vi "Sweep iteration instruction generator with starting step (SubVI).vi"(5 "Sweep plane & fixed axis":string, 6 "Sweep starts later":i32, 7 "Octant":string, 8 "Angle theta [degrees]":dbl, 9 "Magnetic field strength [µT]":dbl, 10 "Number of steps":dbl, 11 "Current iteration":i32) -> (0 "Magnetic field z [µT]":dbl, 1 "Magnetic field y [µT]":dbl, 2 "Magnetic field x [µT]":dbl, 3 "Azimuthal angle \"phi\"":dbl, 4 "Output string instruction":string)   [LabVIEW 2018]
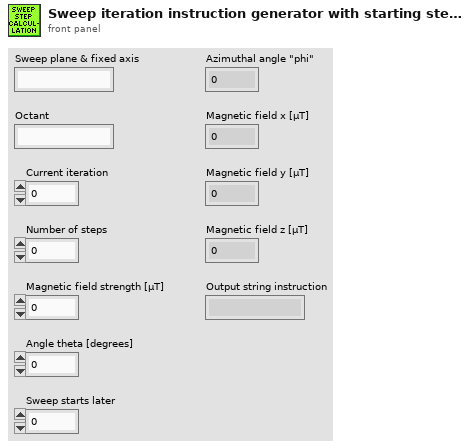
[diagram p1: front panel]
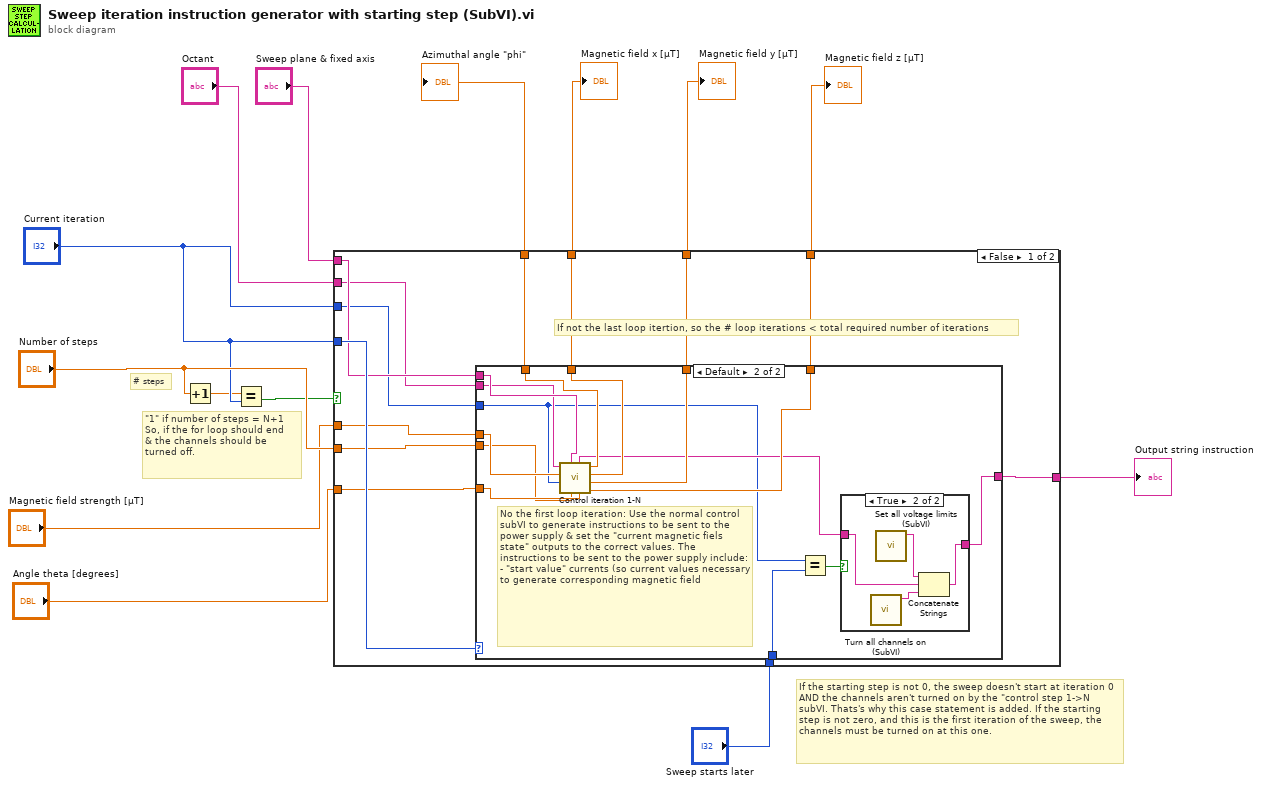
[diagram p0: block diagram]
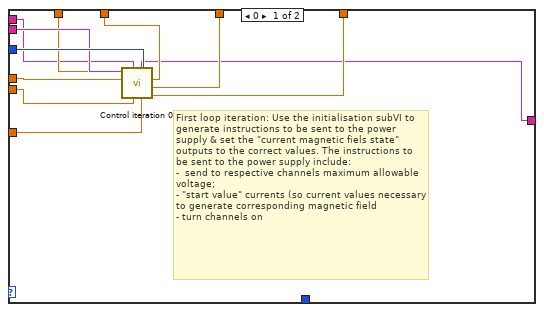
[diagram p2: hidden frame]
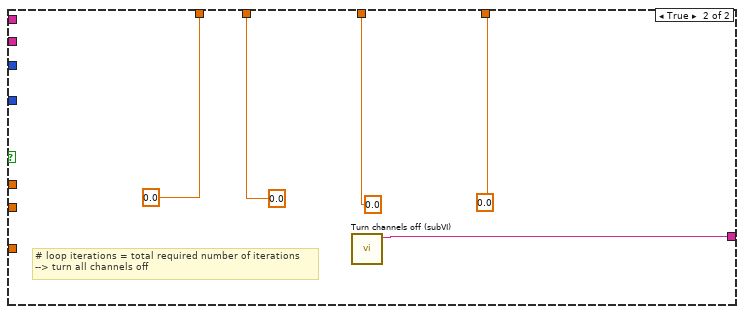
[diagram p4: hidden frame]
diagram:
  # "If the starting step is not 0, the sweep doesn't start at iteration 0 AND the channels aren't turned on by the \"control step 1->N subVI. Thats's why this case statement is added. If the starting step is not zero, and this is the first iteration of the sweep, the channels must be turned on at this one."
  # "\"1\" if number of steps = N+1\nSo, if the for loop should end \n& the channels should be \nturned off."
  # "# steps"
  n1 = Increment(x="Number of steps") -> (x+1=w1:dbl)
  n2 = Equal?(x=w1, y="Current iteration") -> (x = y?=w11:bool)
  n3 = case shown="False" w11 {
    tunnel: [w20 0.0 ("Azimuthal angle \"phi\"")] -> w10
    tunnel: [w17 0.0 ("Magnetic field x [µT]")] -> w6
    tunnel: [w19 0.0 ("Magnetic field y [µT]")] -> w5
    tunnel: [w18 0.0 ("Magnetic field z [µT]")] -> w4
    tunnel: "Current iteration" -> [w27 _]
    tunnel: "Sweep plane & fixed axis" -> [w26 _]
    tunnel: "Octant" -> [w25 _]
    tunnel: "Magnetic field strength [µT]" -> [w24 _]
    tunnel: "Current iteration" -> [w23 _]
    tunnel: "Number of steps" -> [w22 _]
    tunnel: "Angle theta [degrees]" -> [w21 _]
    tunnel: [w16 w58] -> w3
    tunnel: "Sweep starts later" -> [w15 _]
    frame False {
      # "If not the last loop itertion, so the # loop iterations < total required number of iterations"
      n4 = case shown="Default" w27 {
        tunnel: w26 -> [w29 w52]
        tunnel: w25 -> [w33 w51]
        tunnel: w24 -> [w38 w50]
        tunnel: w23 -> [w37 w40]
        tunnel: w22 -> [w28 w44]
        tunnel: w21 -> [w36 w49]
        tunnel: [w30 w48] -> w20
        tunnel: [w32 w47] -> w17
        tunnel: [w34 w46] -> w19
        tunnel: [w35 w45] -> w18
        tunnel: [w31 w41] -> w16
        tunnel: w15 -> [_ w43]
        frame 0 {
          # "First loop iteration: Use the initialisation subVI to generate instructions to be sent to the power supply & set the \"current magnetic fiels state\" outputs to the correct values. The instructions to be sent to the power supply include:\n-  send to respective channels maximum allowable voltage;\n- \"start value\" currents (so current values necessary to generate corresponding magnetic field \n- turn channels on"
          n5 = call "Control iteration 0.vi"("Angle theta [degrees]"=w36, "Number of steps"=w28, "Sweep plane & fixed axis"=w29, "Current iteration"=w37, "Magnetic field strength [µT]"=w38, "Octant"=w33) -> ("Magnetic field z [µT]"=w35:dbl, "Magnetic field y [µT]"=w34:dbl, "Magnetic field x [µT]"=w32:dbl, "Current angle"=w30:dbl, "Output instructions iteration 0"=w31:string)  [unwired: 1 in]
        }
        frame Default {
          # "No the first loop iteration: Use the normal control subVI to generate instructions to be sent to the power supply & set the \"current magnetic fiels state\" outputs to the correct values. The instructions to be sent to the power supply include:\n- \"start value\" currents (so current values necessary to generate corresponding magnetic field"
          n6 = call "Control iteration 1-N.vi"("Angle theta [degrees]"=w49, "Number of steps"=w44, "Sweep plane & fixed axis"=w52, "Current iteration"=w40, "Magnetic field strength [µT]"=w50, "Octant"=w51) -> ("Magnetic field z [µT]"=w45:dbl, "Magnetic field y [µT]"=w46:dbl, "Magnetic field x [µT]"=w47:dbl, "Current angle"=w48:dbl, "Output instructions 1->N"=w42:string)  [unwired: 1 in]
          n7 = Equal?(x=w40, y=w43) -> (x = y?=w39:bool)
          n8 = case shown="True" w39 {
            tunnel: w42 -> [w53 w56]
            tunnel: [w53 w54] -> w41
            frame False {
            }
            frame True {
              n9 = call "Turn all channels on (SubVI).vi"() -> ("String"=w57:string)  [unwired: 11 in]
              n10 = call "Set all voltage limits (SubVI).vi"() -> ("String"=w55:string)  [unwired: 11 in]
              n11 = Concatenate Strings(w55, w56, w57) -> (w54:string)
            }
          }
        }
      }
    }
    frame True {
      # "# loop iterations = total required number of iterations\n--> turn all channels off"
      n12 = call "Turn channels off (subVI).vi"() -> ("String"=w58:string)  [unwired: 11 in]
    }
  }
  "Azimuthal angle \"phi\"" <- w10
  "Magnetic field x [µT]" <- w6
  "Magnetic field y [µT]" <- w5
  "Magnetic field z [µT]" <- w4
  "Output string instruction" <- w3
